vi "Stepper Motor 2.0 Working.vi"() -> ()   [LabVIEW 2017]
uses:
  <vilib>/myRIO/Instrument Drivers/Onboard IO/DIO/typedefs/DIO Reference.ctl
  <vilib>/myRIO/Common/Instrument Driver Framework/Utilities/typedefs/myRIO Generic Hardware Reference.ctl
  <vilib>/myRIO/Common/Instrument Driver Framework/Utilities/typedefs/Hardware Version Enum.ctl
  <vilib>/myRIO/Common/Instrument Driver Framework/Utilities/typedefs/myRIO v1.0 Reference.ctl
  <vilib>/myRIO/Common/Instrument Driver Framework/Utilities/typedefs/Generic FPGA Reference.ctl
  <vilib>/myRIO/Common/Instrument Driver Framework/myRIO v1.0/DIO/typedefs/DIO Channels List.ctl
  <vilib>/myRIO/Common/Instrument Driver Framework/myRIO v1.0/DIO/typedefs/DIO Channels Enum.ctl
  <vilib>/userdefined/High Color/nirio_resource_hc.ctl
  <vilib>/myRIO/Common/Instrument Driver Framework/Utilities/vis/Is FPGA Ref Available.vi
  <vilib>/myRIO/Common/Instrument Driver Framework/myRIO v1.0/DIO/vis/myRIO v1.1 Open DIO.vi
  <vilib>/myRIO/Instrument Drivers/Onboard IO/DIO/vis/Write.vi
  <vilib>/myRIO/Common/Instrument Driver Framework/Utilities/vis/Validate Channels.vi
  <vilib>/myRIO/Common/Instrument Driver Framework/myRIO v1.0/DIO/vis/myRIO v1.0 Reserve DIO.vi
  <vilib>/myRIO/Common/Instrument Driver Framework/myRIO v1.0/Resource Manager/vis/myRIO v1.0 Reserve Channel List.vi
  <vilib>/myRIO/Common/Instrument Driver Framework/myRIO v1.0/DIO/vis/myRIO v1.0 Build MUX Configuration DIO.vi
  <vilib>/myRIO/Common/Instrument Driver Framework/myRIO v1.0/Resource Manager/vis/myRIO v1.0 Reserve Channel.vi
  <vilib>/myRIO/Common/Instrument Driver Framework/myRIO v1.0/Resource Manager/vis/myRIO v1.0 Unreserve Channel.vi
  <vilib>/myRIO/Common/Instrument Driver Framework/myRIO v1.0/Resource Manager/vis/myRIO v1.0 Create Configuration List.vi
  <vilib>/myRIO/Common/Instrument Driver Framework/myRIO v1.0/Resource Manager/vis/myRIO v1.0 Build Mutex Name.vi
  <vilib>/Utility/VariantDataType/GetNumericInfo.vi
  <vilib>/Utility/error.llb/Error Cluster From Error Code.vi
  <vilib>/myRIO/Common/Instrument Driver Framework/myRIO v1.0/myRIO v1.1 Open.vi
  <vilib>/myRIO/Common/Instrument Driver Framework/Utilities/vis/IO Manager.vi
  <vilib>/myRIO/Common/Instrument Driver Framework/Utilities/vis/Configuration Manager.vi
  <vilib>/myRIO/Common/Instrument Driver Framework/myRIO v1.0/Resource Manager/vis/myRIO v1.0 Configure IO.vi
  <vilib>/myRIO/Common/Instrument Driver Framework/myRIO v1.0/myRIO v1.0 Close.vi
  <vilib>/myRIO/Common/Instrument Driver Framework/myRIO v1.0/DIO/vis/myRIO v1.0 Write DIO.vi
  <vilib>/myRIO/Express VI/Onboard Devices/LED/LED Express VI.xnode
  <vilib>/myRIO/Instrument Drivers/Onboard IO/DIO/vis/myRIO DIO Open.xnode
  <vilib>/myRIO/Express VI/Onboard IO/DO/DO Express VI.xnode
  <vilib>/myRIO/Instrument Drivers/Onboard IO/DIO/DIO.lvlib
panel:
  in  "steps/in":dbl
  in  "y (inches)":dbl
  out "current pps d":dbl
  out "loop num d":i32
  out "nc":dbl format="%.2f"
  out "current pps c":dbl
  out "loop num c":i32
  out "na":dbl format="%.2f"
  in  "max pps":dbl
  in  "increment pps":dbl
  out "current pps a":dbl
  out "loop num a":i32
  in  "Dir":bool=TRUE
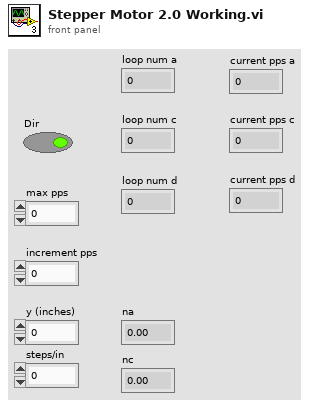
[diagram p1: front panel]
types:
  T1 = typedef "DIO.lvlib/DIO Reference.ctl" = cluster{"myRIO Reference":T2, "DIO Channels List":T6}
  T2 = typedef "myRIO Generic Hardware Reference.ctl" = cluster{"myRIO Model":T3, "myRIO Hardware Reference":T4}
  T3 = typedef "Hardware Version Enum.ctl" = enum16{"Unknown", "myRIO-1900", "myRIO-1950", "roboRIO", "NI ELVIS RIO CM"}
  T4 = typedef "myRIO v1.0 Reference.ctl" = cluster{"Generic FPGA Reference":T5, "Allow multiple opens":bool}
  T5 = typedef "Generic FPGA Reference.ctl" = refnum<k20>
  T6 = typedef "DIO Channels List.ctl" = T7[]
  T7 = typedef "DIO Channels Enum.ctl" = enum16{"Not Connected", "C/DIO0", "C/DIO1", "C/DIO2", "C/DIO3", "C/DIO4", "C/DIO5", "C/DIO6", "C/DIO7", "A/DIO0", "A/DIO1", "A/DIO2", "A/DIO3", "A/DIO4", "A/DIO5", "A/DIO6", "A/DIO7", "A/DIO8", "A/DIO9", "A/DIO10", "A/DIO11", "A/DIO12", "A/DIO13", "A/DIO14", "A/DIO15", "B/DIO0", "B/DIO1", "B/DIO2", "B/DIO3", "B/DIO4", "B/DIO5", "B/DIO6", "B/DIO7", "B/DIO8", "B/DIO9", "B/DIO10", "B/DIO11", "B/DIO12", "B/DIO13", "B/DIO14", "B/DIO15", "LED0", "LED1", "LED2", "LED3", "Button0", "DIO/DIO0", "DIO/DIO1", "DIO/DIO2", "DIO/DIO3", "DIO/DIO4", "DIO/DIO5", "DIO/DIO6", "DIO/DIO7", "DIO/DIO8", "DIO/DIO9", "SPI/CS0", "SPI/CS1", "SPI/CS2", "SPI/CS3", "LED RADIO (Green)", "LED RADIO (Red)", "LED COMM (Green)", "LED COMM (Red)", "LED MODE (Green)", "LED MODE (Red)"}
  T8 = typedef "nirio_resource_hc.ctl" = tag
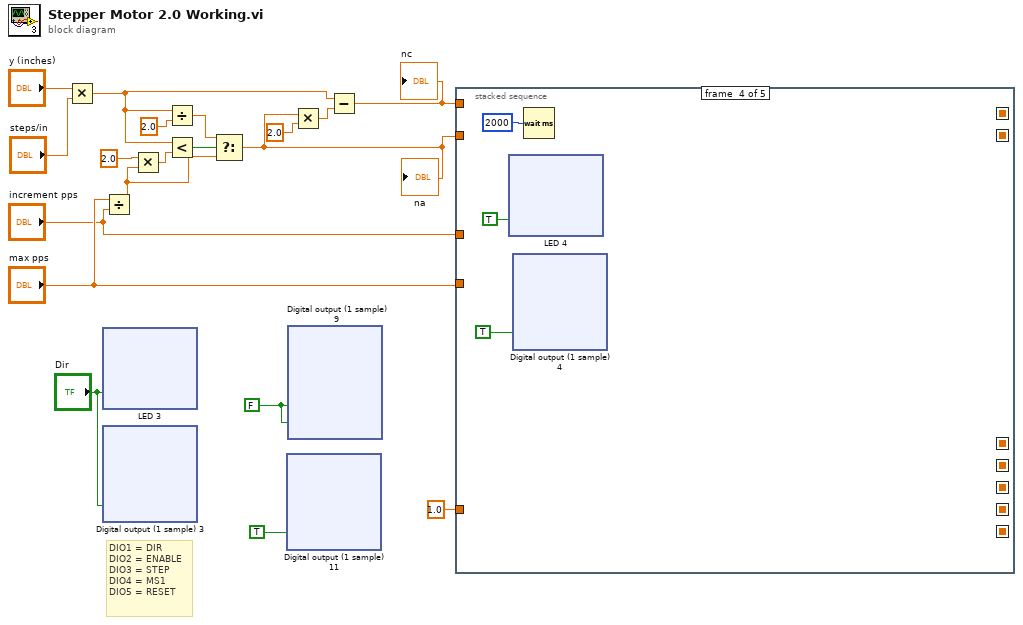
[diagram p0: block diagram]
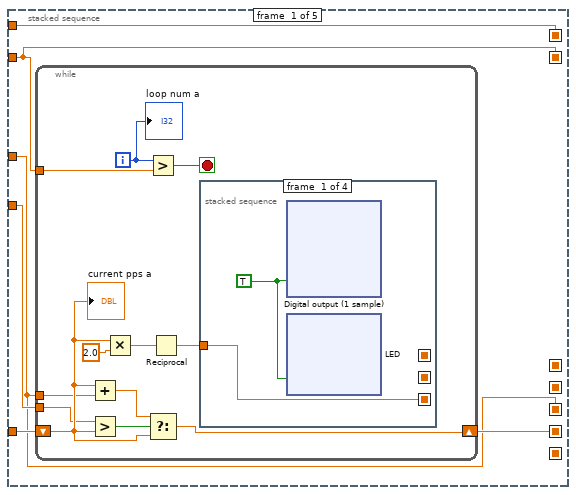
[diagram p2: hidden frame]
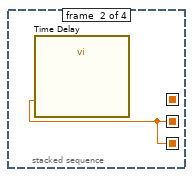
[diagram p3: hidden frame]
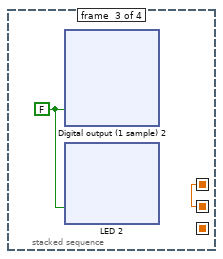
[diagram p4: hidden frame]
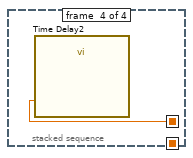
[diagram p5: hidden frame]
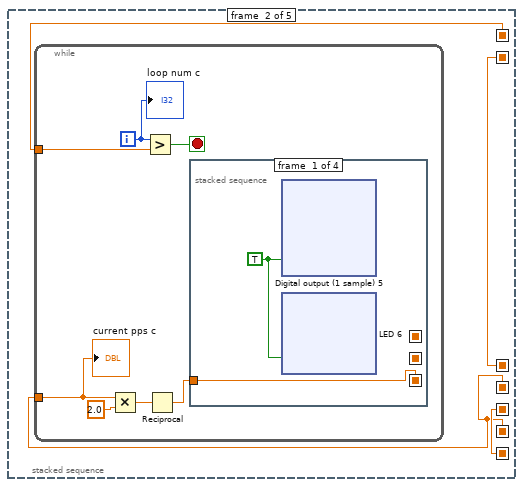
[diagram p6: hidden frame]
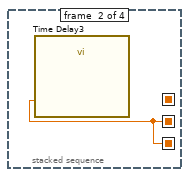
[diagram p7: hidden frame]
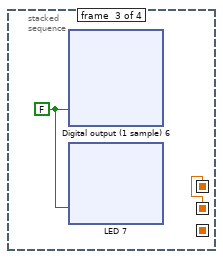
[diagram p8: hidden frame]
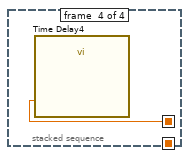
[diagram p9: hidden frame]
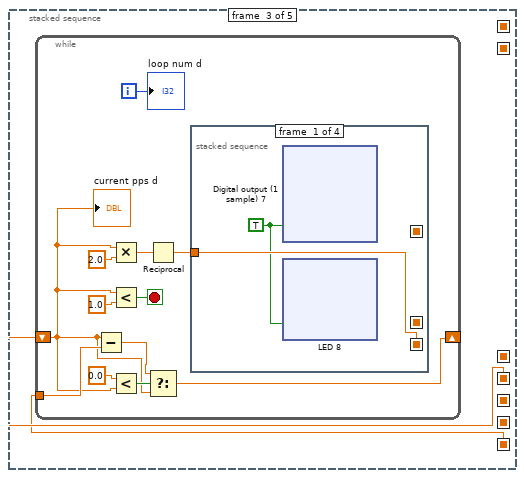
[diagram p10: hidden frame]
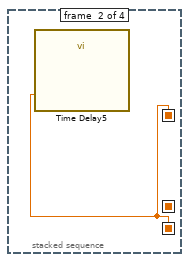
[diagram p11: hidden frame]
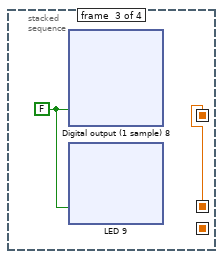
[diagram p12: hidden frame]
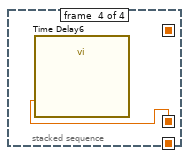
[diagram p13: hidden frame]
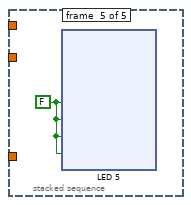
[diagram p14: hidden frame]
diagram:
  w1 = FALSE
  # "DIO1 = DIR\nDIO2 = ENABLE\nDIO3 = STEP\nDIO4 = MS1\nDIO5 = RESET"
  n1 = Multiply(x="y (inches)", y="steps/in") -> (x*y=w6:dbl)
  n2 = xnode "LED 3"("LED0"="Dir") -> ()  [unwired: 1 in, 1 out]
  n3 = xnode "Digital output (1 sample) 3"("DIR (A/DIO1 (Pin 13))"="Dir") -> ()  [unwired: 1 in, 1 out]
  n4 = Divide(x="max pps", y="increment pps") -> (x/y=w3:dbl)
  n5 = Multiply(x=2.0 ("y"), y=w3) -> (x*y=w13:dbl)
  n6 = Divide(x=w6, y=2.0) -> (x/y=w10:dbl)
  n7 = Less?(x=w6, y=w13) -> (x < y?=w12:bool)
  n8 = Select(t=w10, s=w12, f=w3) -> (s? t:f=w7:dbl)
  "na" <- w7
  n9 = xnode "Digital output (1 sample) 11"("A/DIO5 (Pin 21)"=TRUE) -> ()  [unwired: 1 in, 1 out]
  n10 = xnode "Digital output (1 sample) 9"("A/DIO4 (Pin 19)"=w1, "A/DIO2 (Pin 15)"=w1) -> ()  [unwired: 1 in, 1 out]
  n11 = Multiply(x=w7, y=2.0) -> (x*y=w9:dbl)
  n12 = Subtract(x=w6, y=w9) -> (x-y=w5:dbl)
  "nc" <- w5
  n13 = stacked-sequence {
    seq-local: [w23 _ _ _ _] -> [_ w184 _ _ _]
    seq-local: [w22 _ _ _ _] -> [_ w185 _ _ _]
    seq-local: [w21 _ _ _ _] -> [_ w187 _ _ _]
    seq-local: [w20 _ _ _ _] -> [_ w186 _ _ _]
    seq-local: [_ w187 _ _ _] -> [_ _ w341 _ _]
    seq-local: [_ w186 _ _ _] -> [_ _ _ _ _]
    seq-local: [_ w185 _ _ _] -> [_ _ w342 _ _]
    tunnel: "max pps" -> [w25 _ _ _ _]
    tunnel: "increment pps" -> [w21 _ _ _ _]
    tunnel: 1.0 ("starting pps") -> [w24 _ _ _ _]
    tunnel: w7 -> [w20 _ _ _ _]
    tunnel: w5 -> [w23 _ _ _ _]
    frame #0 {
      n14 = while {
        shift-right: [w32] -> w22
        shift-left: w24 -> [w31]
        tunnel: w25 -> [w30]
        tunnel: w21 -> [w29]
        tunnel: w20 -> [w27]
        i -> [w26]
        stop <- w28 stop-if-true
        n15 = Add(x=w31, y=w29) -> (x+y=w33:dbl)
        n16 = Greater?(x=w30, y=w31) -> (0:w34:bool)
        n17 = Multiply(x=w31, y=2.0) -> (x*y=w37:dbl)
        n18 = Greater?(x=w26, y=w27) -> (0:w28:bool)
        n19 = Select(t=w33, s=w34, f=w31) -> (s? t:f=w32:dbl)
        n20 = Reciprocal(x=w37) -> (1/x=w35:dbl)
        n21 = stacked-sequence {
          seq-local: [w39 _ _ _] -> [_ w110 _ _]
          seq-local: [_ w110 _ _] -> [_ _ w112 _]
          seq-local: [_ _ w112 _] -> [_ _ _ w183]
          tunnel: w35 -> [w39 _ _ _]
          frame #0 {
            w38 = TRUE
            n22 = xnode "Digital output (1 sample)"("A/DIO3 (Pin 17)"=w38) -> ()  [unwired: 1 in, 1 out]
            n23 = xnode "LED"("LED1"=w38) -> ()  [unwired: 1 in, 1 out]
          }
          frame #1 {
            n24 = call "Time Delay"("Delay Time (s)"=w110) -> ()  [unwired: 10 in, 1 out]
          }
          frame #2 {
            w111 = FALSE
            n25 = xnode "Digital output (1 sample) 2"("A/DIO3 (Pin 17)"=w111) -> ()  [unwired: 1 in, 1 out]
            n26 = xnode "LED 2"("LED1"=w111) -> ()  [unwired: 1 in, 1 out]
          }
          frame #3 {
            n27 = call "Time Delay2"("Delay Time (s)"=w183) -> ()  [unwired: 10 in, 1 out]
          }
        }
        "current pps a" <- w31
        "loop num a" <- w26
      }
    }
    frame #1 {
      n28 = while {
        tunnel: w184 -> [w189]
        tunnel: w185 -> [w191]
        i -> [w188]
        stop <- w190 stop-if-true
        n29 = Multiply(x=w191, y=2.0) -> (x*y=w194:dbl)
        n30 = Greater?(x=w188, y=w189) -> (0:w190:bool)
        n31 = Reciprocal(x=w194) -> (1/x=w192:dbl)
        n32 = stacked-sequence {
          seq-local: [w196 _ _ _] -> [_ w267 _ _]
          seq-local: [_ w267 _ _] -> [_ _ w269 _]
          seq-local: [_ _ w269 _] -> [_ _ _ w340]
          tunnel: w192 -> [w196 _ _ _]
          frame #0 {
            w195 = TRUE
            n33 = xnode "Digital output (1 sample) 5"("A/DIO3 (Pin 17)"=w195) -> ()  [unwired: 1 in, 1 out]
            n34 = xnode "LED 6"("LED1"=w195) -> ()  [unwired: 1 in, 1 out]
          }
          frame #1 {
            n35 = call "Time Delay3"("Delay Time (s)"=w267) -> ()  [unwired: 10 in, 1 out]
          }
          frame #2 {
            w268 = FALSE
            n36 = xnode "Digital output (1 sample) 6"("A/DIO3 (Pin 17)"=w268) -> ()  [unwired: 1 in, 1 out]
            n37 = xnode "LED 7"("LED1"=w268) -> ()  [unwired: 1 in, 1 out]
          }
          frame #3 {
            n38 = call "Time Delay4"("Delay Time (s)"=w340) -> ()  [unwired: 10 in, 1 out]
          }
        }
        "current pps c" <- w191
        "loop num c" <- w188
      }
    }
    frame #2 {
      n39 = while {
        shift-right: [w346] -> _
        shift-left: w342 -> [w344]
        tunnel: w341 -> [w348]
        i -> [w345]
        stop <- w354 stop-if-true
        n40 = Subtract(x=w344, y=w348) -> (x-y=w350:dbl)
        n41 = Multiply(x=w344, y=2.0) -> (x*y=w353:dbl)
        n42 = Less?(x=w344, y=1.0) -> (x < y?=w354:bool)
        n43 = Less?(x=0.0, y=w344) -> (x < y?=w351:bool)
        n44 = Reciprocal(x=w353) -> (1/x=w349:dbl)
        n45 = Select(t=w350, s=w351, f=w344) -> (s? t:f=w346:dbl)
        n46 = stacked-sequence {
          seq-local: [w356 _ _ _] -> [_ w427 _ _]
          seq-local: [_ w427 _ _] -> [_ _ w429 _]
          seq-local: [_ _ w429 _] -> [_ _ _ w500]
          tunnel: w349 -> [w356 _ _ _]
          frame #0 {
            w355 = TRUE
            n47 = xnode "Digital output (1 sample) 7"("A/DIO3 (Pin 17)"=w355) -> ()  [unwired: 1 in, 1 out]
            n48 = xnode "LED 8"("LED1"=w355) -> ()  [unwired: 1 in, 1 out]
          }
          frame #1 {
            n49 = call "Time Delay5"("Delay Time (s)"=w427) -> ()  [unwired: 10 in, 1 out]
          }
          frame #2 {
            w428 = FALSE
            n50 = xnode "Digital output (1 sample) 8"("A/DIO3 (Pin 17)"=w428) -> ()  [unwired: 1 in, 1 out]
            n51 = xnode "LED 9"("LED1"=w428) -> ()  [unwired: 1 in, 1 out]
          }
          frame #3 {
            n52 = call "Time Delay6"("Delay Time (s)"=w500) -> ()  [unwired: 10 in, 1 out]
          }
        }
        "loop num d" <- w345
        "current pps d" <- w344
      }
    }
    frame #3 {
      n53 = xnode "LED 4"("LED2"=TRUE) -> ()  [unwired: 1 in, 1 out]
      n54 = xnode "Digital output (1 sample) 4"("A/DIO2 (Pin 15)"=TRUE) -> ()  [unwired: 1 in, 1 out]
      n55 = Wait (ms)(milliseconds to wait=u32 2000) -> ()  [unwired: 1 out]
    }
    frame #4 {
      w574 = FALSE
      n56 = xnode "LED 5"("LED0"=w574, "LED1"=w574, "LED2"=w574, "LED3"=w574) -> ()  [unwired: 1 in, 1 out]
    }
  }
